vi "Destroy.vi"(8 "error in (no error)":errorcluster, 11 "Connection in":refnum<class "Connection.lvclass">) -> (0 "error out":errorcluster)   [LabVIEW 2012, in "MDSplus.lvlib" / "Connection.lvclass"]
uses:
  <vilib>/MDSplus/Classes/Connection_Class/Connection.lvclass
  <vilib>/MDSplus/Classes/Connection_Class/Connection.lvclass/Connection.ctl
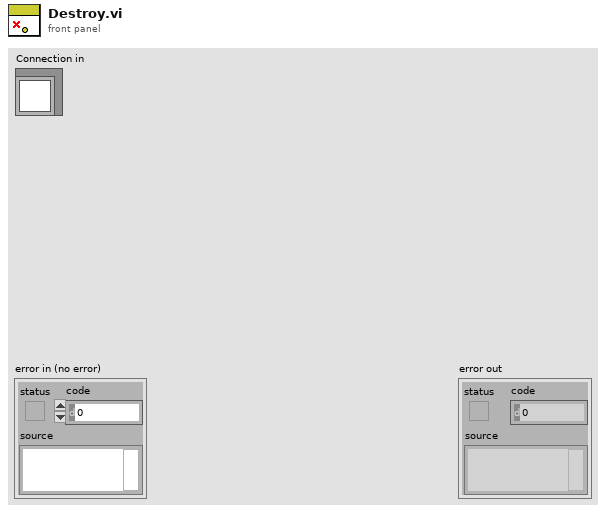
[diagram p1: front panel]
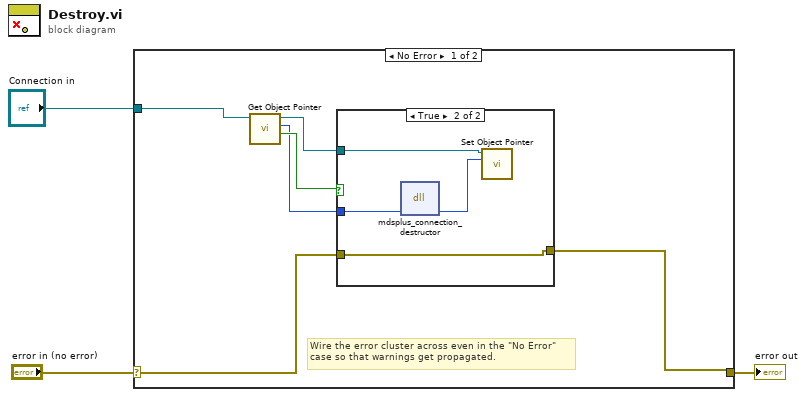
[diagram p0: block diagram]
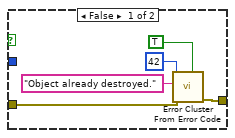
[diagram p2: hidden frame]
diagram:
  n1 = case shown="No Error" "error in (no error)" {
    selector: "error in (no error)" -> [w5 w19]
    tunnel: [w4 w19] -> w2
    tunnel: "Connection in" -> [w9 _]
    frame No Error {
      # "Wire the error cluster across even in the \"No Error\"\ncase so that warnings get propagated."
      n2 = call <vilib>:"Get Object Pointer.vi"("Connection in"=w9) -> ("Assigned object pointer?"=w7:bool, "Object Pointer"=w6:i64, "Connection out"=w8:refnum<class "Connection.lvclass">)  [unwired: 7 in, 1 out]
      n3 = case shown="True" w7 {
        tunnel: [w12 w15] -> w4
        tunnel: w8 -> [_ w18]
        tunnel: w6 -> [_ w16]
        tunnel: w5 -> [w10 w15]
        frame False {
          n4 = call <vilib>:"Error Cluster From Error Code.vi"("is warning? (False)"=TRUE, "error in (no error)"=w10, "error message (\"\")"="Object already destroyed." ("error message (\"\")"), "error code (0)"=42) -> ("error out"=w12:errorcluster)  [unwired: 5 in]
        }
        frame True {
          n5 = dll-call lib="MDSobjectsLVShr" fn="mdsplus_connection_destructor"("lvConnectionPtr"=w16) -> ("lvConnectionPtr"=w17:i64)  [unwired: 4 in, 2 out]
          n6 = call <vilib>:"Set Object Pointer.vi"("Object Pointer"=w17, "Connection in"=w18) -> ()  [unwired: 8 in, 2 out]
        }
      }
    }
    frame Error {
    }
  }
  "error out" <- w2
